vi "DI DAQ.vi"(8 "error in":errorcluster, 11 "All Queue":T1) -> (0 "error out":errorcluster)   [LabVIEW 2022 SP3]
uses:
  Controls/All Queue Ref.ctl
  <vilib>/DAQmx/read.llb/DAQmx Read (Digital 1D Wfm NChan NSamp).vi
  6D_Global.vi
  <vilib>/DAQmx/create/channels.llb/DAQmx Create Channel (DI-Digital Input).vi
  <vilib>/DAQmx/configure/timing.llb/DAQmx Timing (Sample Clock).vi
  <vilib>/DAQmx/configure/trigger.llb/DAQmx Start Trigger (Time).vi
  <vilib>/DAQmx/miscellaneous.llb/DAQmx Fill In Error Info.vi
  <vilib>/Waveform/DWDTOps.llb/DWDT Digital to Boolean Array.vi
  <resource>/objmgr/daqmx.rc
panel:
  in  "DI Data":T2={"DI Config"=[{"DI Signal List"="DI 0", "DI Channel list"="cDAQ9185-1E540F5Mod1/port0/line0", "DI Default Value"=FALSE, "DI Invert"=FALSE}, {"DI Signal List"="DI 1", "DI Channel list"="cDAQ9185-1E540F5Mod1/port0/line1", "DI Default Value"=FALSE, "DI Invert"=FALSE}, {"DI Signal List"="DI 2", "DI Channel list"="cDAQ9185-1E540F5Mod1/port0/line2", "DI Default Value"=FALSE, "DI Invert"=FALSE}], "Digital Input Samples Data"={"Samples per channel"=100, "Sampling Rate"=1000.0, "Sample Mode"=10178, "Source"="OnboardClock", "Active Edge"=10280}} {"Digital Input Samples Data"."Sample Mode" items=["Finite Samples"=10178, "Continuous Samples"=10123, "Hardware Timed Single Point"=12522]; "Digital Input Samples Data"."Active Edge" items=["Rising"=10280, "Falling"=10171]}
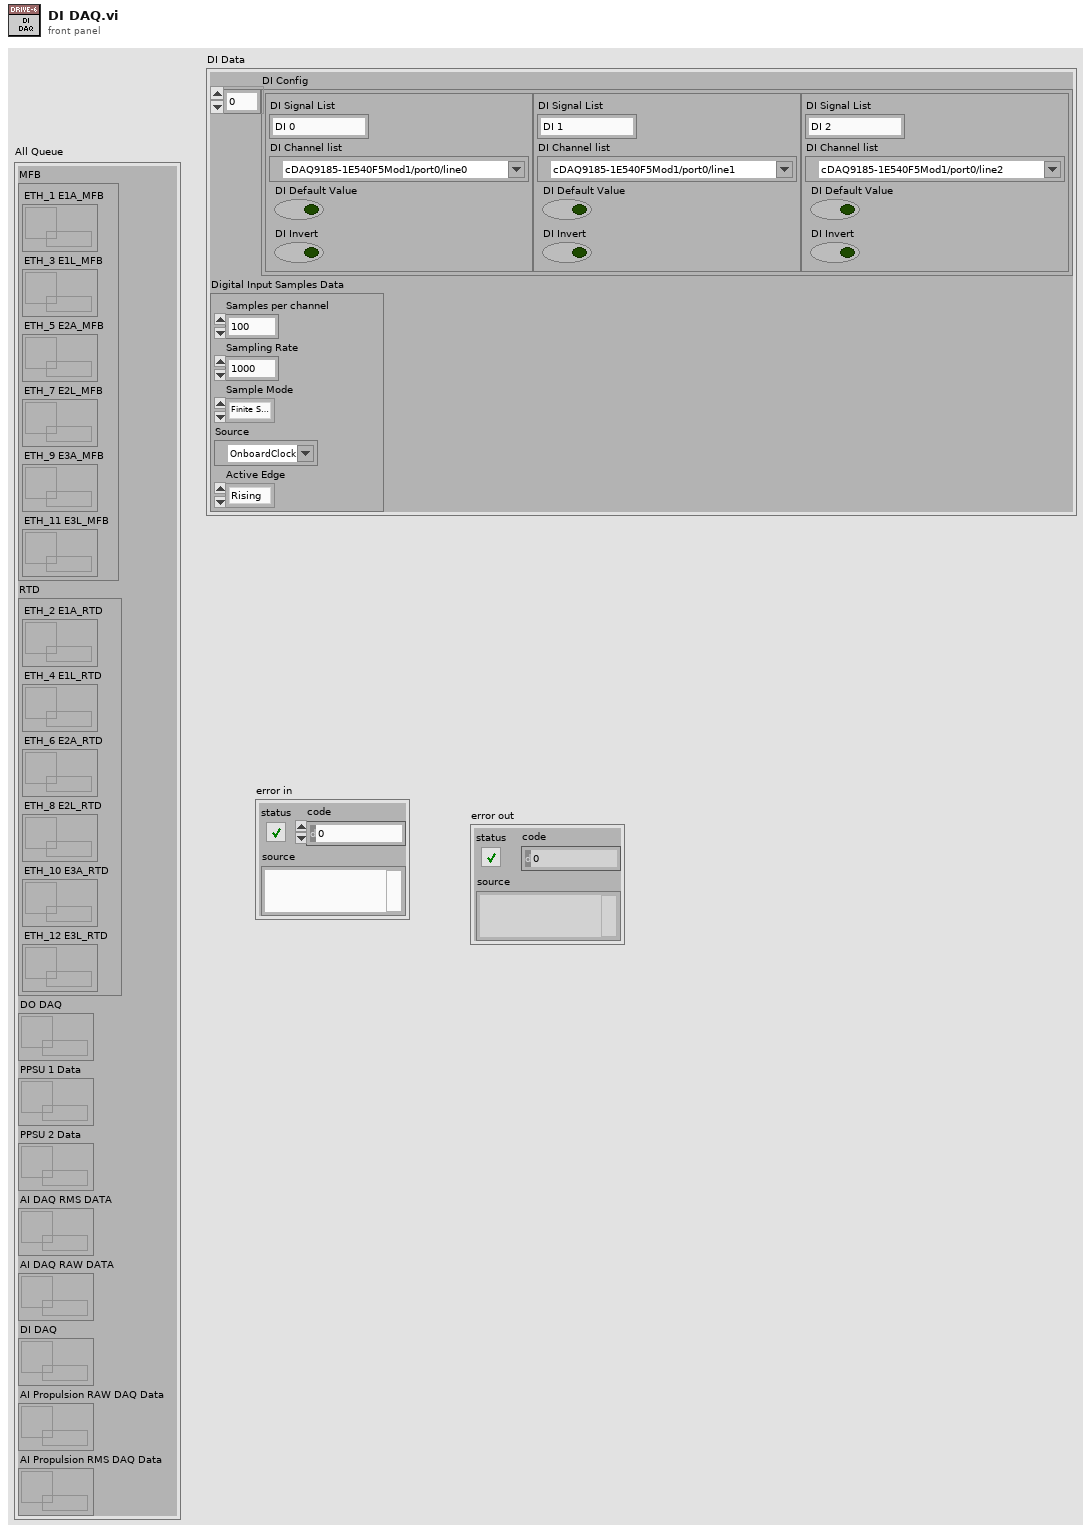
[diagram p1: front panel]
types:
  T1 = typedef "All Queue Ref.ctl" = cluster{"MFB":cluster{"ETH_1 E1A_MFB":refnum<queue>, "ETH_3 E1L_MFB":refnum<queue>, "ETH_5 E2A_MFB":refnum<queue>, "ETH_7 E2L_MFB":refnum<queue>, "ETH_9 E3A_MFB":refnum<queue>, "ETH_11 E3L_MFB":refnum<queue>}, "RTD":cluster{"ETH_2 E1A_RTD ":refnum<queue>, "ETH_4 E1L_RTD ":refnum<queue>, "ETH_6 E2A_RTD ":refnum<queue>, "ETH_8 E2L_RTD ":refnum<queue>, "ETH_10 E3A_RTD ":refnum<queue>, "ETH_12 E3L_RTD ":refnum<queue>}, "DO DAQ":refnum<queue>, "PPSU 1 Data":refnum<queue>, "PPSU 2 Data":refnum<queue>, "AI DAQ RMS DATA":refnum<queue>, "AI DAQ RAW DATA":refnum<queue>, "DI DAQ":refnum<queue>, "AI Propulsion RAW DAQ Data":refnum<queue>, "AI Propulsion RMS DAQ Data":refnum<queue>}
  T2 = cluster{"DI Config":cluster{"DI Signal List":string, "DI Channel list":tag, "DI Default Value":bool, "DI Invert":bool}[], "Digital Input Samples Data":cluster{"Samples per channel":i32, "Sampling Rate":dbl, "Sample Mode":i32, "Source":tag, "Active Edge":i32}}
  T3 = enum16{"Channel Data Input", "Sampling Data Input", "Read Data", "Stop DAQ"}
  T4 = cluster{"DI Signal List":string, "DI Channel list":tag, "DI Default Value":bool, "DI Invert":bool}[]
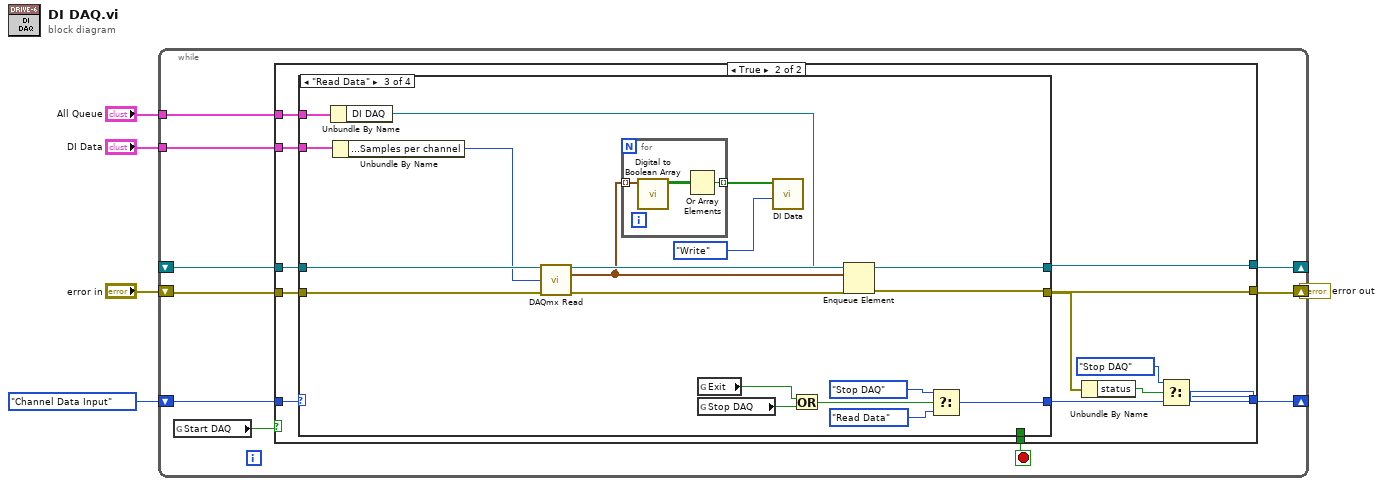
[diagram p0: block diagram]
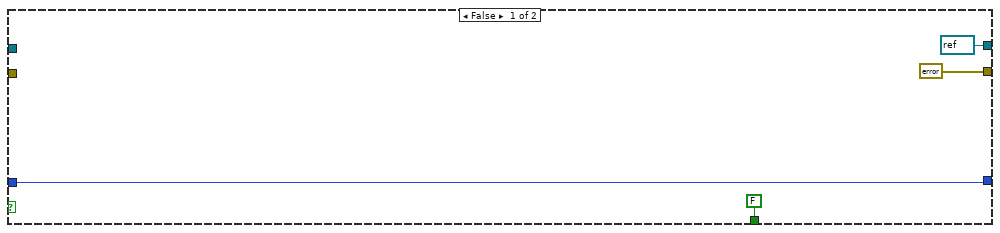
[diagram p2: hidden frame]
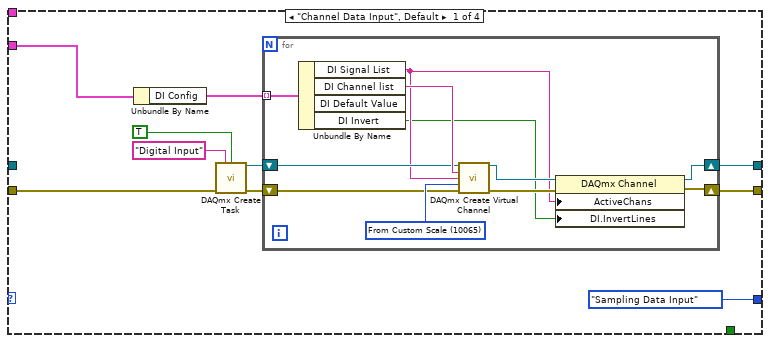
[diagram p3: hidden frame]
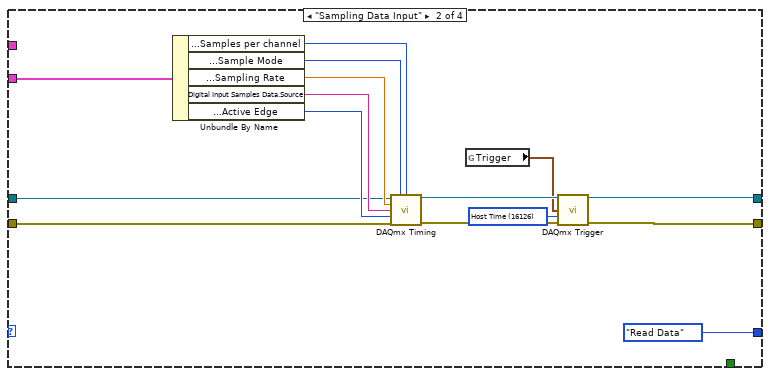
[diagram p4: hidden frame]
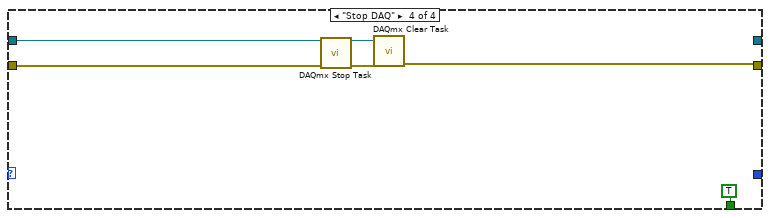
[diagram p5: hidden frame]
diagram:
  n1 = while {
    shift-right: [w11] -> _
    shift-left: T3."Channel Data Input" -> [w15]
    shift-right: [w14] -> _
    shift-left: _ -> [w13]
    shift-right: [w9] -> w5
    shift-left: "error in" -> [w10]
    tunnel: "DI Data" -> [w8]
    tunnel: "All Queue" -> [w6]
    stop <- w12 stop-if-true
    n2 = global read "6D_Global.vi" "Start DAQ"() -> (w7:bool)
    n3 = case shown="True" w7 {
      tunnel: w15 -> [w16 w31]
      tunnel: [refnum<k21> refnum ("task out") w30] -> w14
      tunnel: w13 -> [_ w29]
      tunnel: [FALSE w28] -> w12
      tunnel: [w16 w26] -> w11
      tunnel: w10 -> [_ w24]
      tunnel: [errorcluster {"status"=FALSE, "code"=0, "source"=""} ("error out") w23] -> w9
      tunnel: w8 -> [_ w22]
      tunnel: w6 -> [_ w20]
      frame False {
      }
      frame True {
        n4 = case shown="\"Read Data\"" w31 {
          tunnel: w24 -> [w35 w59 w80 w93]
          tunnel: [w36 w57 w72 w89] -> w23
          tunnel: [w39 w55 w82 _] -> w30
          tunnel: w29 -> [_ w61 w81 w91]
          tunnel: [T3."Sampling Data Input" T3."Read Data" w83 _] -> w27
          tunnel: [_ _ _ TRUE] -> w28
          tunnel: w22 -> [w32 w58 w78 _]
          tunnel: w20 -> [_ _ w74 _]
          frame "Channel Data Input", Default {
            n5 = Unbundle By Name(w32) -> ("DI Config"=w33:T4)
            n6 = call <vilib>:"DAQmx Create Task.vi"("new task name"="Digital Input", "auto cleanup"=TRUE, "error in"=w35) -> ("task out"=w41:refnum<k21>, "error out"=w37:errorcluster)  [unwired: 11 in]
            n7 = for {
              tunnel: w33 -> [w52] mode=indexing
              shift-right: [w45] -> w39
              shift-left: w41 -> [w49]
              shift-right: [w47] -> w36
              shift-left: w37 -> [w42]
              w50 = 10065 items=["Volts"=10348, "From Custom Scale"=10065] ("units")
              n8 = Unbundle By Name(w52) -> ("DI Signal List"=w44:string, "DI Channel list"=w51:tag, "DI Invert"=w43:bool)  [unwired: 1 out]
              n9 = call-poly <vilib>:"DAQmx Create Virtual Channel.vi"("task in"=w49, "lines"=w51, "name to assign"=w44, "line grouping"=w50, "error in"=w42) -> ("task out"=w46:refnum<k21>, "error out"=w48:errorcluster)  [unwired: 9 in]
              n10 = property class="DAQmx Channel"(reference=w46, error in=w48, "ActiveChans"=w44, "DI.InvertLines"=w43) -> (reference out=w45:refnum<k21>, error out=w47:errorcluster)
            }
          }
          frame "Sampling Data Input" {
            w54 = 16126 items=["Host Time"=16126, "I/O Device Time"=16127] ("timescale")
            n11 = Unbundle By Name(w58) -> ("Digital Input Samples Data.Samples per channel"=w63:i32, "Digital Input Samples Data.Sample Mode"=w64:i32, "Digital Input Samples Data.Sampling Rate"=w65:dbl, "Digital Input Samples Data.Source"=w66:tag, "Digital Input Samples Data.Active Edge"=w67:i32)
            n12 = call-poly <vilib>:"DAQmx Timing.vi"("task/channels in"=w61, "sample mode"=w64, "samples per channel"=w63, "rate"=w65, "source"=w66, "active edge"=w67, "error in"=w59) -> ("task out"=w56:refnum<k21>, "error out"=w62:errorcluster)  [unwired: 7 in]
            n13 = global read "6D_Global.vi" "Trigger"() -> (w53:timestamp)
            n14 = call-poly <vilib>:"DAQmx Trigger.vi"("task/channels in"=w56, "when"=w53, "timescale"=w54, "error in"=w62) -> ("task out"=w55:refnum<k21>, "error out"=w57:errorcluster)  [unwired: 10 in]
          }
          frame "Read Data" {
            n15 = Unbundle By Name(w74) -> ("DI DAQ"=w71:refnum<queue>)
            n16 = Unbundle By Name(w78) -> ("Digital Input Samples Data.Samples per channel"=w77:i32)
            n17 = call-poly <vilib>:"DAQmx Read.vi"("task/channels in"=w81, "number of samples per channel"=w77, "error in"=w80) -> ("task out"=w82:refnum<k21>, "data"=w70:digitalwaveform[], "error out"=w73:errorcluster)  [unwired: 10 in]
            n18 = for {
              tunnel: w70 -> [w87] mode=indexing
              tunnel: [w86] -> w69 mode=indexing
              n19 = call-poly <vilib>:"Digital to Boolean Array.vi"("digital waveform"=w87) -> ("boolean array"=w88:bool[][])  [unwired: 9 in, 1 out]
              n20 = Or Array Elements(Boolean array=w88) -> (logical OR=w86:bool)
            }
            n21 = global read "6D_Global.vi" "Exit"() -> (w76:bool)
            n22 = global read "6D_Global.vi" "Stop DAQ"() -> (w75:bool)
            n23 = call "DI Data.vi"("Enum"=enum16{"Write", "Read"}."Write", "DI Data"=w69) -> ()  [unwired: 9 in, 1 out]
            n24 = Or(x=w76, y=w75) -> (x .or. y?=w79:bool)
            n25 = Enqueue Element(queue=w71, element=w70, error in (no error)=w73) -> (error out=w72:errorcluster)  [unwired: 1 in, 2 out]
            n26 = Select(t=T3."Stop DAQ", s=w79, f=T3."Read Data") -> (s? t:f=w83:T3)
          }
          frame "Stop DAQ" {
            n27 = call <vilib>:"DAQmx Stop Task.vi"("task/channels in"=w91, "error in"=w93) -> ("task out"=w90:refnum<k21>, "error out"=w92:errorcluster)  [unwired: 12 in]
            n28 = call <vilib>:"DAQmx Clear Task.vi"("task in"=w90, "error in"=w92) -> ("error out"=w89:errorcluster)  [unwired: 13 in]
          }
        }
        n29 = Unbundle By Name(w23) -> ("status"=w21:bool)
        n30 = Select(t=T3."Stop DAQ", s=w21, f=w27) -> (s? t:f=w26:T3)
      }
    }
  }
  "error out" <- w5
